vi "Decimate (multiple).vi"(8 "error in (no error)":errorcluster, 9 "averaging (off)":bool, 10 "decimating factor (1)":i32=1, 11 "XY-data":cluster{"X-array":dbl[], "Y-array":dbl[]}[](array[cluster]) {"Y-array" format="%.2p"; "X-array" format="%.2p"}) -> (0 "error out":errorcluster, 3 "Decimated XY-data out":cluster{"X-array":dbl[], "Y-array":dbl[]}[](array[cluster]) {"Y-array" format="%.2p"; "X-array" format="%.2p"})   [LabVIEW 2019, in "xy_utilities.lvlib"]
doc: "Decimates the X and Y arrays from the input <b>XY-data</b> by the <b>decimating factor</b> and the <b>averaging</b> Boolean control. \n\nWire data to the data input to determine the polymorphic instance to use or manually select the instance."
uses:
  xy_utilities.lvlib
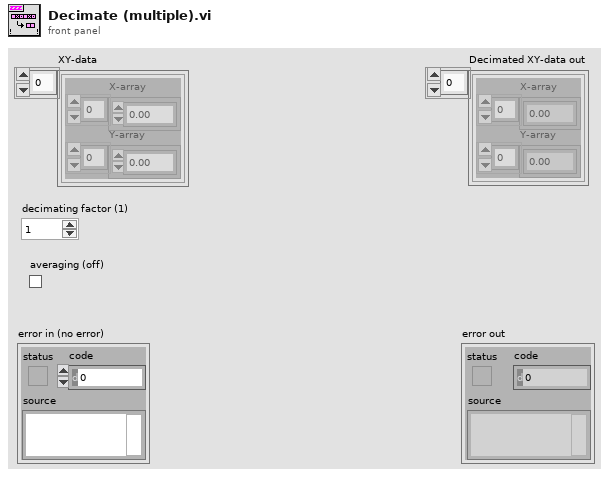
[diagram p1: front panel]
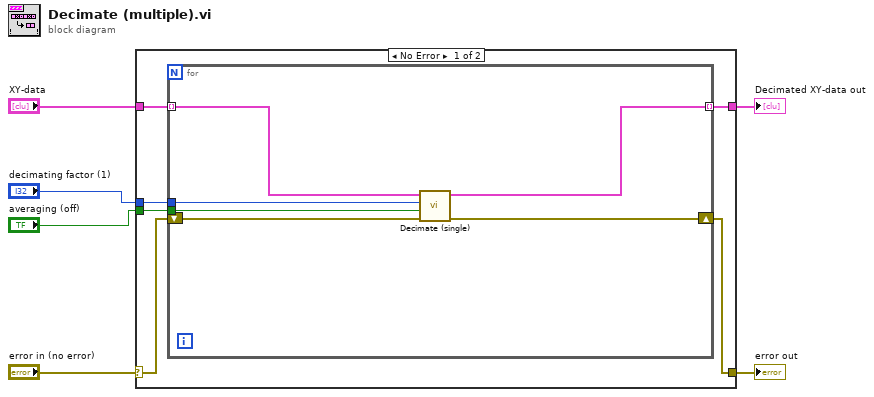
[diagram p0: block diagram]
diagram:
  n1 = case shown="No Error" "error in (no error)" {
    selector: "error in (no error)" -> [w10 w20]
    tunnel: "XY-data" -> [w12 w19]
    tunnel: [w11 w19] -> w4
    tunnel: [w9 w20] -> w3
    tunnel: "decimating factor (1)" -> [w8 _]
    tunnel: "averaging (off)" -> [w7 _]
    frame No Error {
      n2 = for {
        tunnel: w12 -> [w18] mode=indexing
        tunnel: [w17] -> w11 mode=indexing
        shift-right: [w15] -> w9
        shift-left: w10 -> [w16]
        tunnel: w8 -> [w14]
        tunnel: w7 -> [w13]
        n3 = call "Decimate (single).vi"("error in (no error)"=w16, "averaging (off)"=w13, "decimating factor (1)"=w14, "XY-data"=w18) -> ("error out"=w15:errorcluster, "Decimated XY-data out"=w17:cluster{"X-array":dbl[], "Y-array":dbl[]})  [unwired: 6 in]
      }
    }
    frame Error {
    }
  }
  "error out" <- w3
  "Decimated XY-data out" <- w4
